vi "Configure Output Power.vi"(8 "error in (no error)":errorcluster, 10 "Output Power [dBm]":dbl, 11 "SigGen-8665B in":refnum<class "SigGen-8665B.lvclass">) -> (0 "error out":errorcluster, 3 "SigGen-8665B out":refnum<class "SigGen-8665B.lvclass">)   [LabVIEW 2020, in "SigGen-8665B.lvclass"]
uses:
  SigGen-8665B.lvclass
  C:/Sandbox/Git_Sandbox/WiSpry Test Framework source code (LV20)/WiSpry Test Framework/Instruments/Signal Generator/Signal Generator.lvclass
  C:/Sandbox/Git_Sandbox/WiSpry Test Framework source code (LV20)/WiSpry Test Framework/Instruments/Instrument.lvclass
  Signal Generator.lvclass/Signal Generator.ctl
  Instrument.lvclass/Instrument.ctl
  Signal Generator.lvclass
  Instrument.lvclass
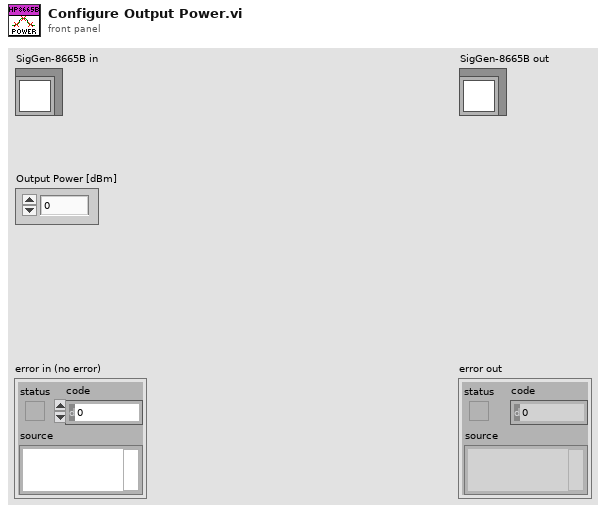
[diagram p1: front panel]
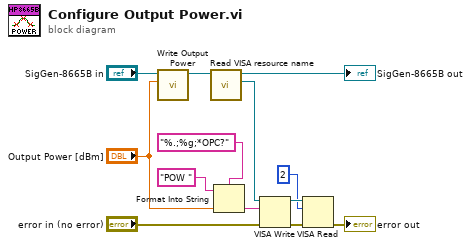
[diagram p0: block diagram]
diagram:
  n1 = call "Write Output Power.vi"("Output Power"="Output Power [dBm]", "Signal Generator in"="SigGen-8665B in") -> ("Signal Generator out"=w12:refnum<class "SigGen-8665B.lvclass">)  [unwired: 9 in]
  n2 = call "Read VISA resource name.vi"("Instrument in"=w12) -> ("VISA resource name"=w8:refnum<visa-resource-name>, "Instrument out"=→"SigGen-8665B out":refnum<class "SigGen-8665B.lvclass">)  [unwired: 9 in]
  n3 = Format Into String(format string="%.;%g;*OPC?", initial string="POW ", "Output Power [dBm]") -> (resulting string=w1:string)  [unwired: 1 in, 1 out]
  n4 = VISA Write(VISA resource name=w8, write buffer=w1, error in (no error)="error in (no error)") -> (VISA resource name out=w5:refnum<visa-resource-name>, error out=w6:errorcluster)  [unwired: 1 out]
  n5 = VISA Read(VISA resource name=w5, byte count=u32 2, error in (no error)=w6) -> (error out=→"error out":errorcluster)  [unwired: 3 out]
